vi "Validate Receive Times Increasing.vi"(8 "error in (no error)":errorcluster, 10 "receive times":dbl[](array[numeric]), 11 "CAN Loopback Tests in":refnum<class "CAN Loopback Tests.lvclass">) -> (0 "error out":errorcluster, 3 "CAN Loopback Tests out":refnum<class "CAN Loopback Tests.lvclass">)   [LabVIEW 2017, in "CAN Loopback Tests.lvclass"]
uses:
  CAN Loopback Tests.lvclass
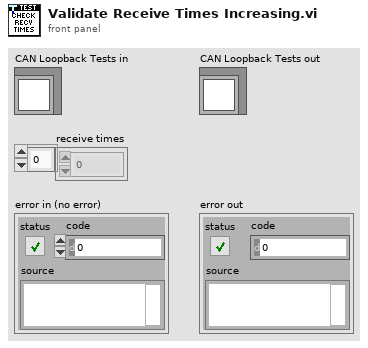
[diagram p1: front panel]
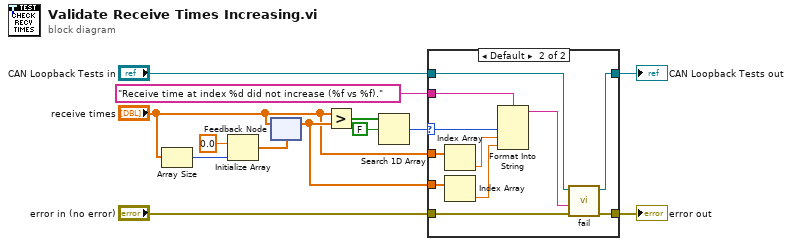
[diagram p0: block diagram]
diagram:
  n1 = Array Size(array="receive times") -> (size(s)=w13:i32)
  n2 = Initialize Array(0.0 ("element"), w13) -> (w12:dbl[])
  n3 = feedback-in #1("receive times") -> ()
  n4 = feedback #1(w12) -> (w2:dbl[])
  n5 = Greater?(x="receive times", y=w2) -> (0:w10:bool[])
  n6 = Search 1D Array(1D array=w10, element=FALSE) -> (index of element=w8:i32)  [unwired: 1 in]
  n7 = case shown="Default" w8 {
    selector: w8 -> [_ w22]
    tunnel: "error in (no error)" -> [w14 w26]
    tunnel: [w14 w25] -> w6
    tunnel: "CAN Loopback Tests in" -> [w15 w24]
    tunnel: [w15 w23] -> w4
    tunnel: "Receive time at index %d did not increase (%f vs %f)." ("format string") -> [_ w20]
    tunnel: w2 -> [_ w18]
    tunnel: "receive times" -> [_ w19]
    frame -1 {
    }
    frame Default {
      n8 = Index Array(array=w19) -> (element=w17:dbl)  [unwired: 1 in]
      n9 = Index Array(array=w18) -> (element=w16:dbl)  [unwired: 1 in]
      n10 = Format Into String(format string=w20, w22, w17, w16) -> (resulting string=w21:string)  [unwired: 2 in, 1 out]
      n11 = call-dynamic "fail.vi"("error in (no error)"=w26, "message (\"\")"=w21, "TestCase in"=w24) -> ("error out"=w25:errorcluster, "TestCase out"=w23:refnum<class "CAN Loopback Tests.lvclass">)  [unwired: 7 in]
    }
  }
  "CAN Loopback Tests out" <- w4
  "error out" <- w6
